vi "Set_IP_Simulation_Duration .vi"(8 "error in (no error)":errorcluster, 9 "Cellular Technology":T1="2G", 10 "Value":string, 11 "Base Station":T2) -> (0 "error out":errorcluster, 3 "Output String":string)   [LabVIEW 2021]
uses:
  Controls/Base_Station_Emulator.ctl
  Controls/Cellular_Technology.ctl
  Controls/TCP_FGV.ctl
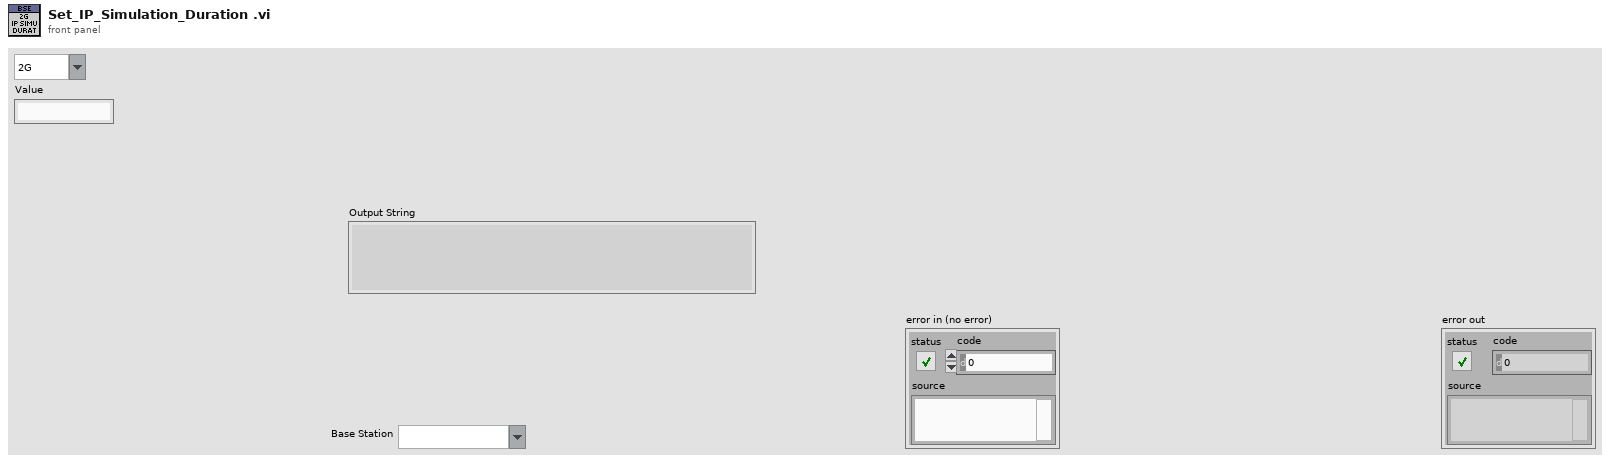
[diagram p1: front panel]
types:
  T1 = typedef "Cellular_Technology.ctl" = string
  T2 = typedef "Base_Station_Emulator.ctl" = string
  T3 = typedef "TCP_FGV.ctl" = enum16{"Open", "Read", "Write", "Close"}
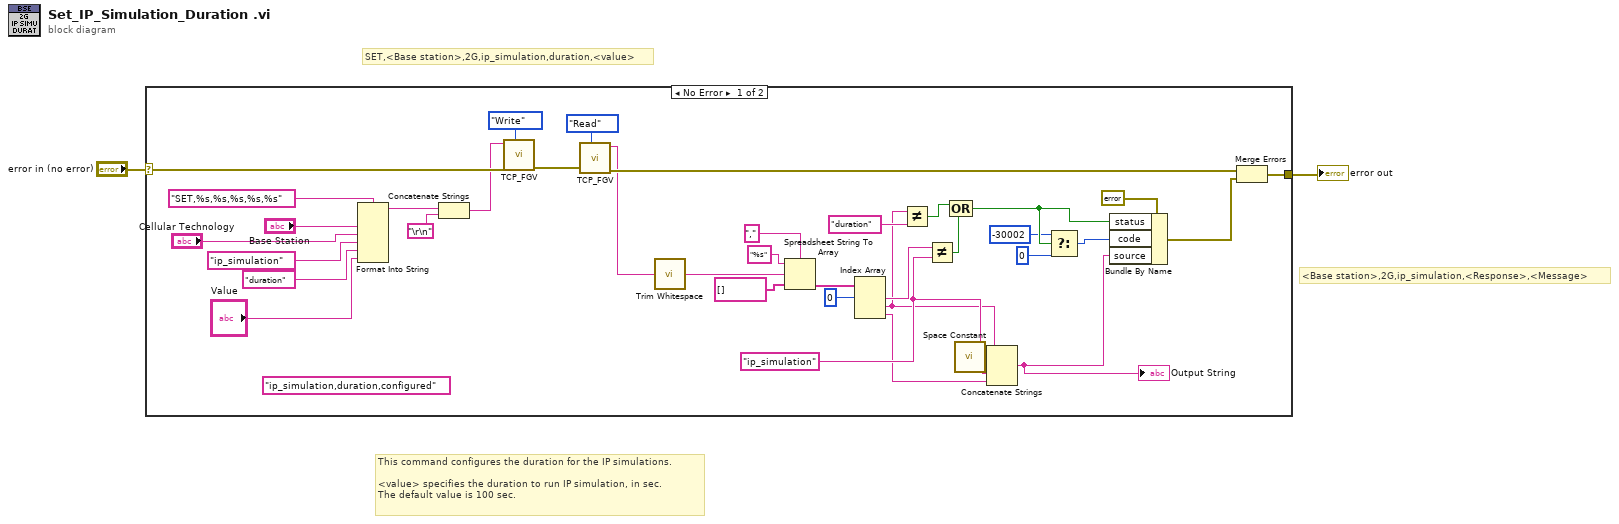
[diagram p0: block diagram]
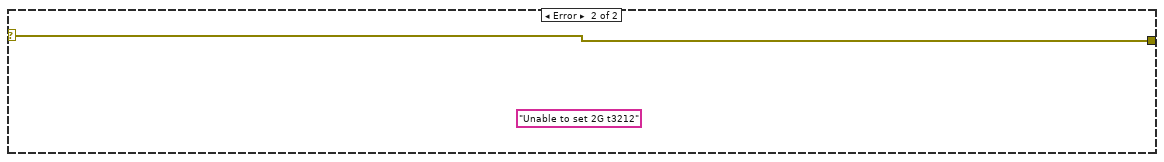
[diagram p2: hidden frame]
diagram:
  # "<Base station>,2G,ip_simulation,<Response>,<Message>"
  # "This command configures the duration for the IP simulations.\n \n<value> specifies the duration to run IP simulation, in sec. \nThe default value is 100 sec."
  # "SET,<Base station>,2G,ip_simulation,duration,<value>"
  n1 = case shown="No Error" "error in (no error)" {
    selector: "error in (no error)" -> [w36 w40]
    tunnel: [w19 w40] -> w1
    frame No Error {
      (unwired) "ip_simulation,duration,configured" ("format string")
      w10 = "ip_simulation" ("format string")
      n2 = Format Into String(format string="SET,%s,%s,%s,%s,%s", "Base Station", "Cellular Technology", "ip_simulation", "duration", "Value") -> (resulting string=w14:string)  [unwired: 2 in, 1 out]
      n3 = Concatenate Strings(w14, "\r\n") -> (w13:string)
      n4 = call "TCP_FGV.vi"("Command"=w13, "error in (no error)"=w36, "Operation"=TCP_FGV."Write") -> ("error out"=w20:errorcluster)  [unwired: 6 in, 1 out]
      n5 = call "TCP_FGV.vi"("error in (no error)"=w20, "Operation"=TCP_FGV."Read") -> ("Data Out"=w7:string, "error out"=w22:errorcluster)  [unwired: 7 in]
      n6 = call <vilib>:"Trim Whitespace.vi"("string"=w7) -> ("trimmed string"=w33:string)  [unwired: 1 in]
      n7 = Spreadsheet String To Array(delimiter (Tab)=",", format string="%s", spreadsheet string=w33, array type (2D Dbl)=string[] []) -> (array=w30:string[])
      n8 = Index Array(array=w30, index #1=0 ("index")) -> (element #1=w23:string, element #2=w4:string, element #3=w8:string)  [unwired: 2 in]
      n9 = Not Equal?(x=w4, y="duration") -> (x != y?=w31:bool)
      n10 = Not Equal?(x=w23, y=w10) -> (x != y?=w32:bool)
      n11 = Compound Arithmetic op=OR(w31, w32) -> (w34:bool)
      n12 = call <vilib>:"Space Constant.vi"() -> ("String"=w9:string)
      n13 = Concatenate Strings(w10, w9, w4, w9, w8) -> (w18:string)
      "Output String" <- w18
      n14 = Select(t=-30002 ("code"), s=w34, f=0 ("code")) -> (s? t:f=w35:i32)
      n15 = Bundle By Name(cluster=errorcluster {"status"=FALSE, "code"=0, "source"=""} ("error constant"), "status"=w34, "code"=w35, "source"=w18) -> (w21:errorcluster)
      n16 = Merge Errors(w22, w21) -> (w19:errorcluster)
    }
    frame Error {
      (unwired) "Unable to set 2G t3212" ("source")
    }
  }
  "error out" <- w1
